vi "Module Cleanup.vi"(8 "error in (no error)":errorcluster, 11 "Data Logger Module in":refnum<class "Data Logger DBL Module.lvclass">) -> (0 "error out":errorcluster, 3 "Data Logger Module out":refnum<class "Data Logger DBL Module.lvclass">)   [LabVIEW 2020, in "VolatusData.lvlib" / "Data Logger DBL Module.lvclass"]
uses:
  Data Logger DBL Module.lvclass
  Volatus/MessageQ/MessageQ.lvclass
  Unregister Logger.ctl
  VolatusData.lvlib
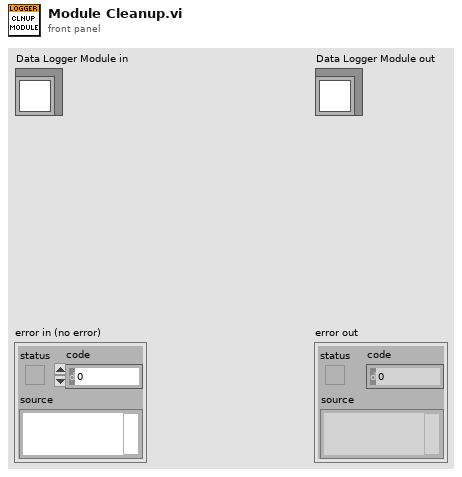
[diagram p1: front panel]
types:
  T1 = typedef "VolatusData.lvlib/Unregister Logger.ctl" = cluster{"ID":string}
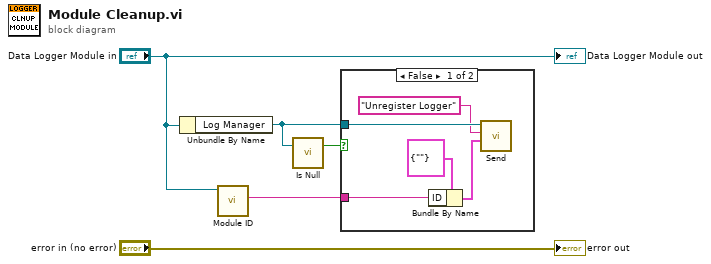
[diagram p0: block diagram]
diagram:
  n1 = Unbundle By Name("Data Logger Module in") -> ("Log Manager"=w3:refnum<class "MessageQ.lvclass">)
  n2 = call-dynamic "Module ID.vi"("Data Logger Module in"="Data Logger Module in") -> ("Module ID"=w1:string)  [unwired: 10 in]
  n3 = call "Is Null.vi"("MessageQ in"=w3) -> ("Null"=w4:bool)  [unwired: 2 in]
  n4 = case shown="False" w4 {
    tunnel: w3 -> [w10 _]
    tunnel: w1 -> [w7 _]
    frame False {
      n5 = Bundle By Name(cluster=T1 {"ID"=""} ("Unregister Logger"), "ID"=w7) -> (w6:T1)
      n6 = call "Send.vi"("Data"=w6, "ID"="Unregister Logger", "MessageQ in"=w10) -> ()  [unwired: 7 in, 2 out]
    }
    frame True {
    }
  }
  "error out" <- "error in (no error)"
  "Data Logger Module out" <- "Data Logger Module in"
